vi "SaveConfig.vi"(8 "error in (no error)":errorcluster, 11 "GRMActor in":refnum<class "FlatFieldUI.lvclass">) -> (0 "error out":errorcluster, 3 "GRMActor out":refnum<class "FlatFieldUI.lvclass">)   [LabVIEW 2020, in "FlatFieldUI.lvlib" / "FlatFieldUI.lvclass"]
uses:
  FlatFieldUI.lvclass
  FlatFieldUI.lvclass/FlatFieldUI.ctl
  Hardware Abstraction Layer/Component/GenericActor/GenericActor/GenericController.lvclass
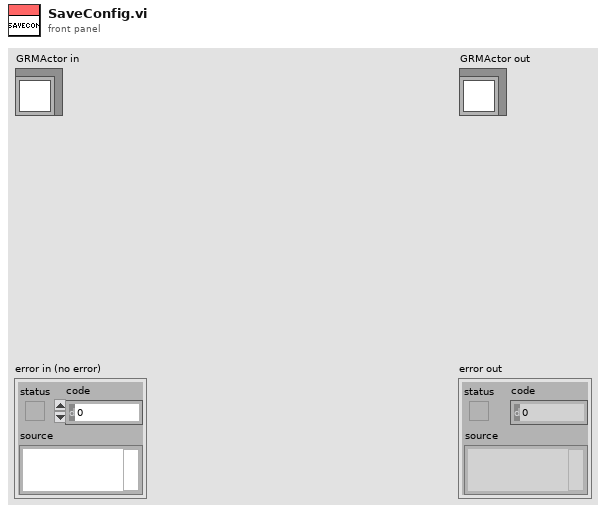
[diagram p1: front panel]
types:
  T1 = typedef "FlatFieldUI.lvlib/FlatFieldUI.lvclass/FlatField Method.ctl" = i32
  T2 = typedef "NI_LVConfig.lvlib/Config Data RefNum.ctl" = refnum<k1>
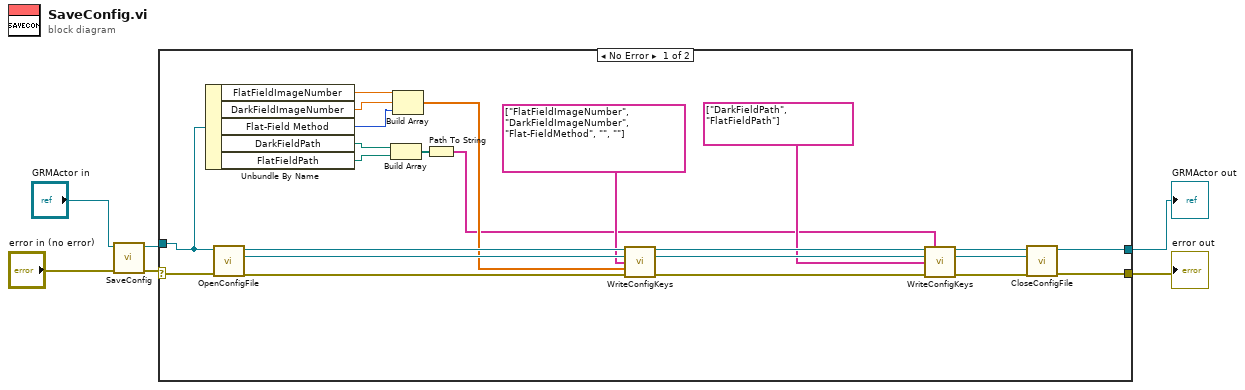
[diagram p0: block diagram]
diagram:
  n1 = call-parent "SaveConfig.vi"("error in (no error)"="error in (no error)", "GRMActor in"="GRMActor in") -> ("error out"=w3:errorcluster, "GRMActor out"=w4:refnum<class "FlatFieldUI.lvclass">)  [unwired: 8 in]
  n2 = case shown="No Error" w3 {
    selector: w3 -> [w29 w30]
    tunnel: [w24 w30] -> w1
    tunnel: [w23 w31] -> w2
    tunnel: w4 -> [w15 w31]
    frame No Error {
      n3 = Unbundle By Name(w15) -> ("FlatFieldImageNumber"=w12:dbl, "DarkFieldImageNumber"=w11:dbl, "Flat-Field Method"=w10:T1, "DarkFieldPath"=w14:path, "FlatFieldPath"=w13:path)
      n4 = call-dynamic "OpenConfigFile.vi"("error in (no error)"=w29, "GRMActor in"=w15) -> ("error out"=w28:errorcluster, "refnum"=w25:T2, "GRMActor out"=w26:refnum<class "FlatFieldUI.lvclass">)  [unwired: 7 in]
      n5 = Build Array(w14, w13) -> (w8:path[])
      n6 = Build Array(w12, w11, w10) -> (w9:dbl[])
      n7 = Path To String(path=w8) -> (string=w7:string[])
      n8 = call-dynamic "WriteConfigKeys.vi"("GRMActor in"=w26, "Config Refnum"=w25, "Keys"=string[] ["FlatFieldImageNumber", "DarkFieldImageNumber", "Flat-FieldMethod", "", ""] ("Values"), "DoubleValue"=w9, "error in (no error)"=w28) -> ("GRMActor out"=w20:refnum<class "FlatFieldUI.lvclass">, "Config Refnum dup"=w18:T2, "error out"=w27:errorcluster)  [unwired: 8 in]
      n9 = call-dynamic "WriteConfigKeys.vi"("GRMActor in"=w20, "StringValues"=w7, "Config Refnum"=w18, "Keys"=string[] ["DarkFieldPath", "FlatFieldPath"], "error in (no error)"=w27) -> ("GRMActor out"=w19:refnum<class "FlatFieldUI.lvclass">, "Config Refnum dup"=w17:T2, "error out"=w21:errorcluster)  [unwired: 8 in]
      n10 = call-dynamic "CloseConfigFile.vi"("error in (no error)"=w21, "refnum"=w17, "GRMActor in"=w19) -> ("error out"=w24:errorcluster, "GRMActor out"=w23:refnum<class "FlatFieldUI.lvclass">)  [unwired: 7 in]
    }
    frame Error {
    }
  }
  "error out" <- w1
  "GRMActor out" <- w2
